vi "Periodic Tasks.vi"(8 "error in":errorcluster) -> ()   [LabVIEW 2018]
doc: "This VI runs in parallel to other tasks. It can contain as many user-defined periodic loops as you need. These can carry out PID or other sorts of timed response."
uses:
  <vilib>/Platform/TimedLoop/XDataNode/timing_clust.ctl
  <vilib>/Platform/TimedLoop/XDataNode/nitl_modes.ctl
  <vilib>/Platform/TimedLoop/XDataNode/wakeup.ctl
  <vilib>/Rock Robotics/WPI/ThirdParty/Phoenix-LabVIEW/Motor Controller/Controls/CTRE_Phoenix_MotorControl_ControlMode.ctl
  <vilib>/Rock Robotics/WPI/Utilities/WPI_GetSetVariantRefNum.vi
  <vilib>/Rock Robotics/WPI/Joystick/WPI_JoystickArcadeMapping.vi
  <vilib>/addons/control/pid/pid.llb/PID (DBL).vi
  <vilib>/addons/control/pid/pid.llb/PID Output Rate Limiter (DBL).vi
  <vilib>/platform/TimedLoop/XDataNode/XDataNode.xnode
  <vilib>/addons/control/pid/NI_PID_pid.lvlib
  <vilib>/Platform/TimedLoop/XDataNode/XDNodeRunTimeDep.lvlib
panel:
  in  "ms to wait":u32=50
  in  "Tab Control":enum32{"Auto Tape Alignment", "Drive PID Tune"}(tab)
  out "Late?":bool
  out "Arrived":bool
  in  "Tol (cnts)":dbl=10.0
  in  "Tol (sec)":dbl=0.25 format="%#_13g"
  in  "Approach":dbl=0.55 format="%#_13g"
  out "Value 1":bool
  out "Value 2":bool
  out "Value 4":bool
  in  "PID gains":T1={"proportional gain (Kc)"=0.005, "integral time (Ti, min)"=0.007, "derivative time (Td, min)"=0.001} {"derivative time (Td, min)" format="%.3f"; "integral time (Ti, min)" format="%.3f"; "proportional gain (Kc)" format="%.3f"}
  in  "clamp":cluster{"output high":dbl, "output low":dbl}={"output high"=0.8, "output low"=-0.8} {"output low" format="%.2f"; "output high" format="%.2f"}
  in  "Fwd offset":dbl=190.0
  in  "Rvs offset":dbl=150.0
  out "Goal":dbl=712.25
  out "Distance":dbl=364.5
  in  "rate":dbl=500.0 format="%.2f"
  out "Tape Width":dbl=34.5
  out "State":i32
  out "Error":dbl=347.75
  out "Align Assist":bool
  in  "Set":dbl(slide)=1.5948963317384823 scale=-1000.0..1000.0
  in  "output range":cluster{"output high":dbl, "output low":dbl}={"output high"=0.8, "output low"=-0.8} {"output low" format="%.2f"; "output high" format="%.2f"}
  in  "PID gains 2":T1={"proportional gain (Kc)"=0.005, "integral time (Ti, min)"=0.007, "derivative time (Td, min)"=0.001} {"derivative time (Td, min)" format="%.3f"; "integral time (Ti, min)" format="%.3f"; "proportional gain (Kc)" format="%.3f"}
  out "PID":cluster{"Set":dbl, "Distance":dbl}(graph)={"Set"=-687.4003189792663, "Distance"=-688.5}
  in  "output rate (EGU/min)":dbl=100.0 format="%.2f"
  out "Distance 2":dbl=-688.5
  out "Error 2":dbl=1.0996810207336694
  out "Motor":dbl=0.010401644622641346 format="%.2f"
  in  "Reset":bool
  in  "reinitialize? (F)":bool
  in  "negate":bool=TRUE
  out "Arrived 2":bool=TRUE
  in  "Tol 2":dbl=10.0
  # "Larger values move goal\nfurther in direction of travel"
  # "2016 Bot values:\nP=0.005, I=0.007, D=0.001"
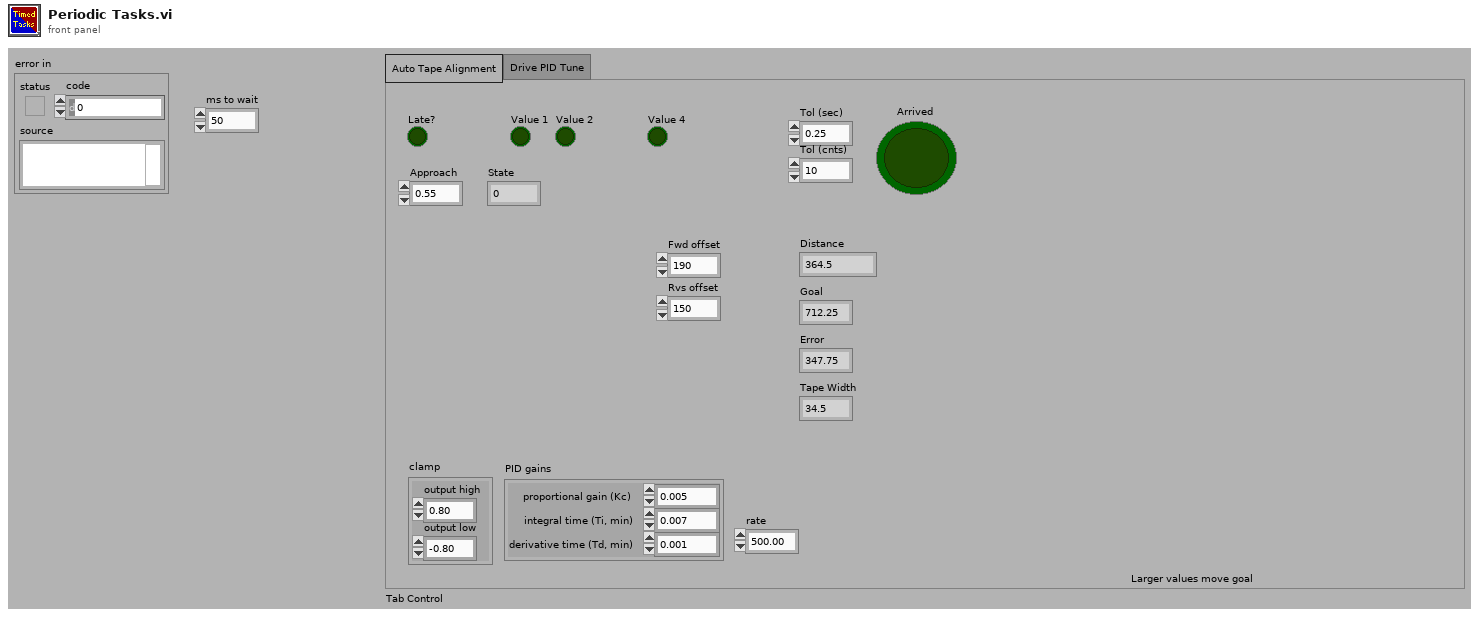
[diagram p1: front panel]
types:
  T1 = cluster{"proportional gain (Kc)":dbl, "integral time (Ti, min)":dbl, "derivative time (Td, min)":dbl}
  T2 = typedef "WPI_EncoderDevRef.ctl" = cluster{"DevStatus":errorcluster, "EncoderIndex":T3, "CounterIndex":T4, "DistancePerCount":dbl, "Decoding Type":T5}
  T3 = typedef "FPGA_EncoderIdx.ctl" = enum8{"Enc 0", "Enc 1", "Enc 2", "Enc 3", "Enc 4", "Enc 5", "Enc 6", "Enc 7", "Invalid"}
  T4 = typedef "FPGA_CounterCtrSystemIndex.ctl" = enum8{"Ctr 0", "Ctr 1", "Ctr 2", "Ctr 3", "Ctr 4", "Ctr 5", "Ctr 6", "Ctr 7", "Invalid"}
  T5 = typedef "WPI_EncoderType.ctl" = enum16{"1x", "2x", "4x"}
  T6 = typedef "WPI_DigitalInputDevRef.ctl" = cluster{"DevStatus":errorcluster, "DIO Channel":T7}
  T7 = typedef "FPGA_DIOChannel.ctl" = enum8{"DIO 0", "DIO 1", "DIO 2", "DIO 3", "DIO 4", "DIO 5", "DIO 6", "DIO 7", "DIO 8", "DIO 9", "DIO MXP 0", "DIO MXP 1", "DIO MXP 2", "DIO MXP 3", "DIO MXP 4", "DIO MXP 5", "DIO MXP 6", "DIO MXP 7", "DIO MXP 8", "DIO MXP 9", "DIO MXP 10", "DIO MXP 11", "DIO MXP 12", "DIO MXP 13", "DIO MXP 14", "DIO MXP 15", "SPI Port CS1", "SPI Port CS2", "SPI Port CS3", "SPI Port MISO", "SPI Port MOSI", "Invalid"}
  T8 = typedef "WPI_MotorControlDeviceRef.ctl" = cluster{"DeviceStatus":errorcluster, "Type":T9, "PWM":cluster{"PWM Channel":T10, "DeadBand":T11}, "CAN":cluster{"Device Number":u8, "SetOutput VI Ref":variant, "GetOutput VI Ref":variant, "Enable VI Ref":variant, "Disable VI Ref":variant, "Data":variant}, "Invert":bool, "DIO PWM":cluster{"PWM \"Enable\" Channel":T10, "DIOChannel":T7, "PWM Rate":dbl}}
  T9 = typedef "WPI_MotorControlType.ctl" = enum16{"PWM", "CAN", "DIO PWM"}
  T10 = typedef "FPGA_DIOPWMChannel.ctl" = enum8{"PWM 0", "PWM 1", "PWM 2", "PWM 3", "PWM 4", "PWM 5", "PWM 6", "PWM 7", "PWM 8", "PWM 9", "PWM MXP 0", "PWM MXP 1", "PWM MXP 2", "PWM MXP 3", "PWM MXP 4", "PWM MXP 5", "PWM MXP 6", "PWM MXP 7", "PWM MXP 8", "PWM MXP 9", "Invalid"}
  T11 = typedef "WPI_PWMDeadband.ctl" = cluster{"Name":string, "maxPositivePwm":i32, "minPositivePwm":i32, "centerPwm":i32, "maxNegativePwm":i32, "minNegativePwm":i32, "angularRange":u16}
  T12 = typedef "WPI_JoystickDevRef.ctl" = cluster{"Device":T13}
  T13 = typedef "WPI_JoystickDeviceEnum.ctl" = enum16{"USB 0", "USB 1", "USB 2", "USB 3", "USB 4", "USB 5"}
  T14 = typedef "XDNodeRunTimeDep.lvlib/timing_clust.ctl" = cluster{"Expected End [f-1]":u64, "Actual End [f-1]":u64, "Finished Late? [f-1]":bool, "Expected End [i-1]":u64, "Actual End [i-1]":u64, "Finished Late? [i-1]":bool, "Expected Start [i]":u64, "Actual Start [i]":u64, "Expected Start [f]":u64, "Actual Start [f]":u64, "Source Name":string, "Structure Name":string, "Period":i64, "Deadline":i64, "Offset":i64, "Start":i64, "Priority":i32, "Timeout":i32, "Mode":T15, "Wakeup Reason":T16, "Error":errorcluster, "Source Type":string, "Secondary Source Type":string, "Global End Time":u64, "Global Start Time":u64, "Frame Duration":u64, "Iteration Duration":u64, "Assigned CPU":i32, "I/O Scan Engine Mode":u32}
  T15 = typedef "XDNodeRunTimeDep.lvlib/nitl_modes.ctl" = enum32{"No Change", "Process missed periods, maintain original phase", "Discard missed periods, maintain original phase", "Process missed periods, ignore original phase", "Discard missed periods, ignore original phase"}
  T16 = typedef "XDNodeRunTimeDep.lvlib/wakeup.ctl" = enum32{"Normal", "Aborted", "Asynchronous wakeup", "Timing source error", "Timed loop error", "Timeout"}
  T17 = typedef "CTRE_Phoenix_MotorControl_ControlMode.ctl" = u16
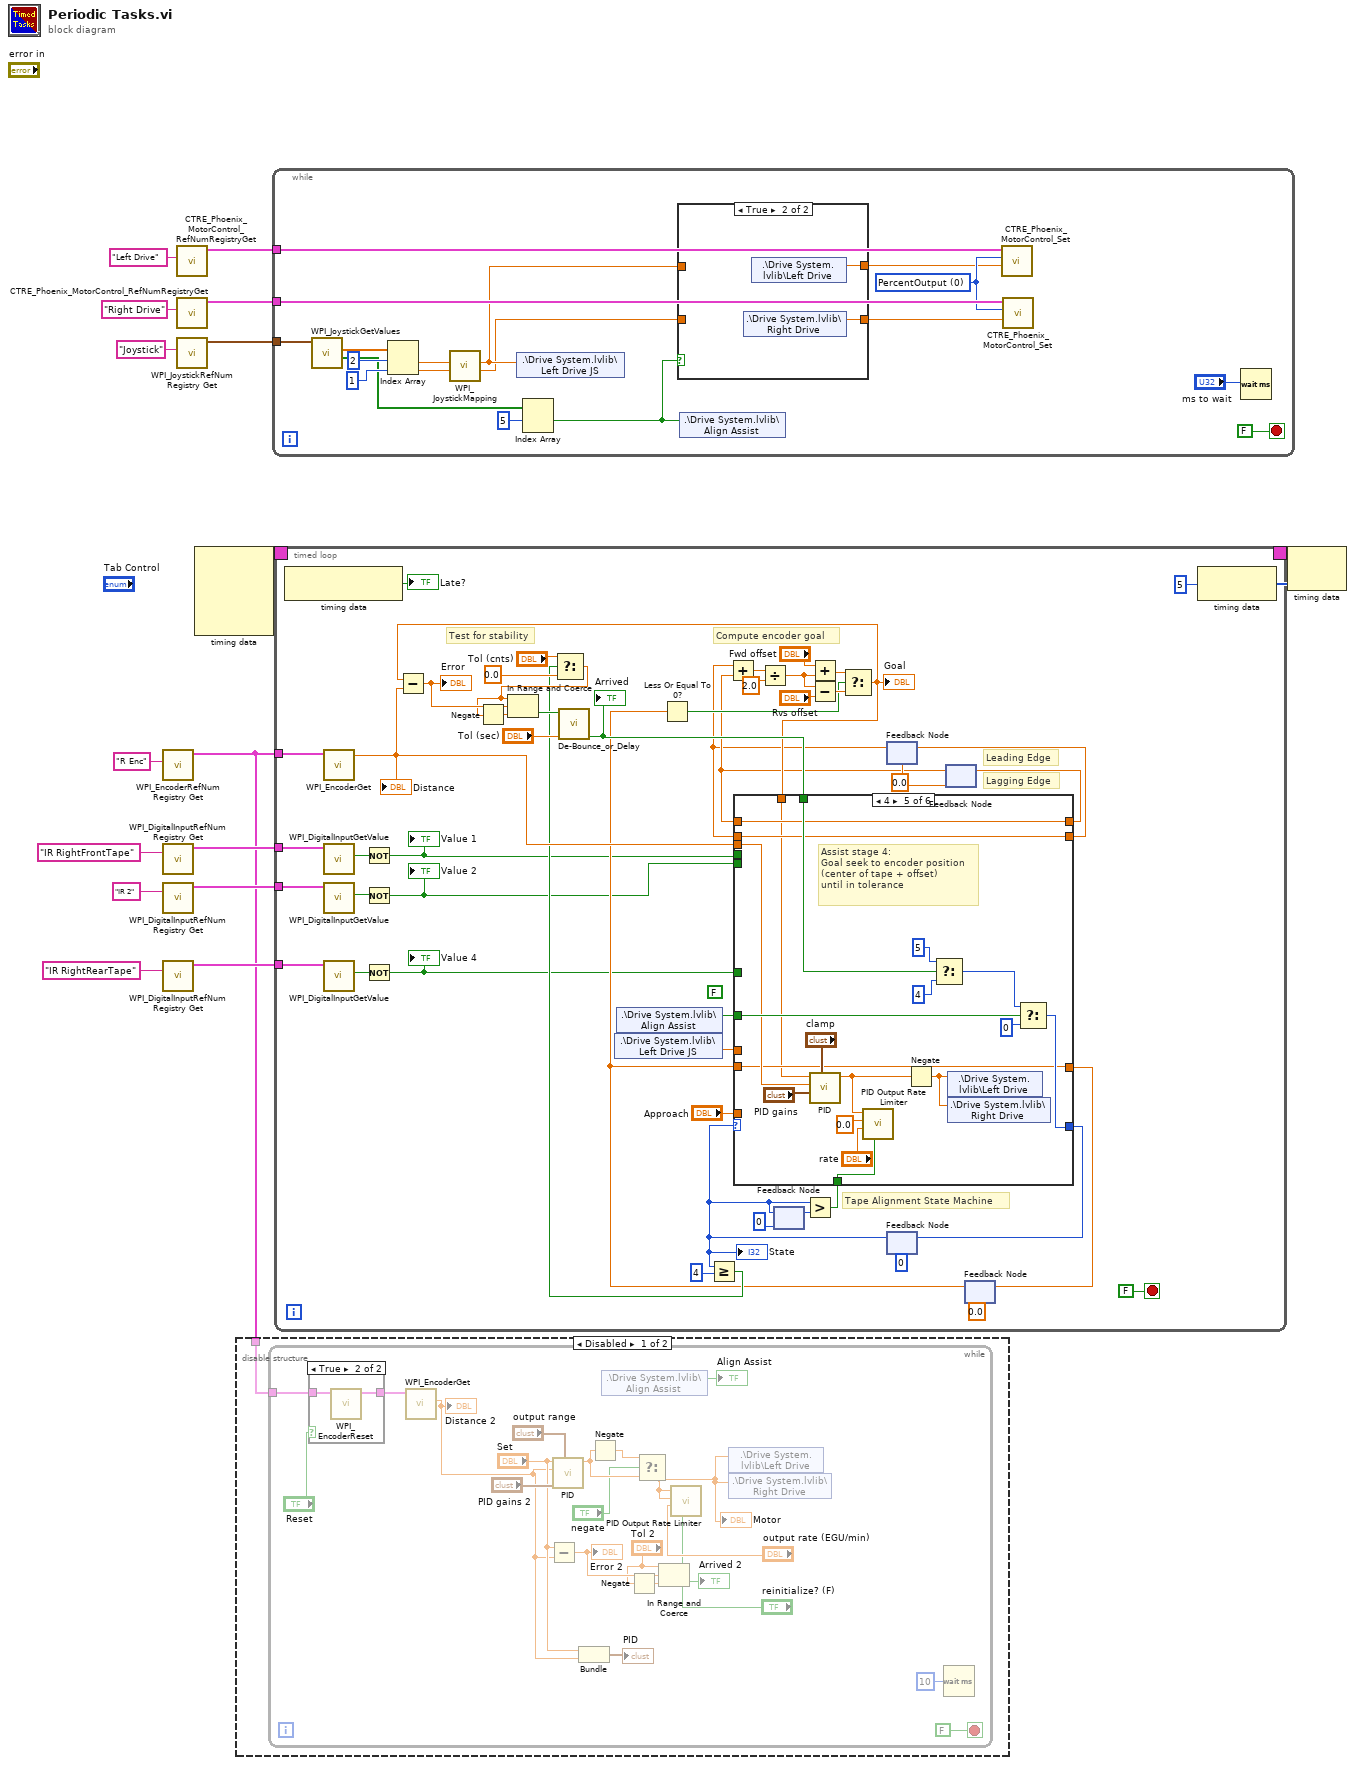
[diagram p0: block diagram]
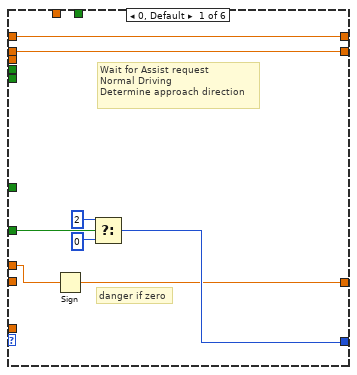
[diagram p2: hidden frame]
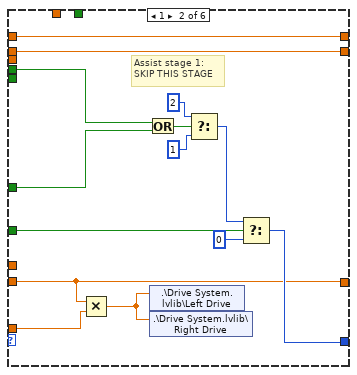
[diagram p3: hidden frame]
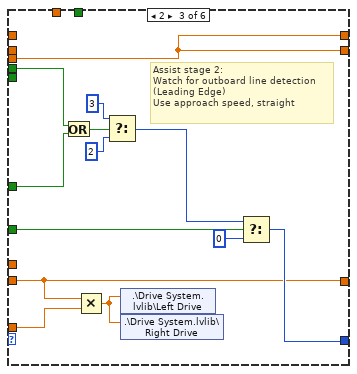
[diagram p4: hidden frame]
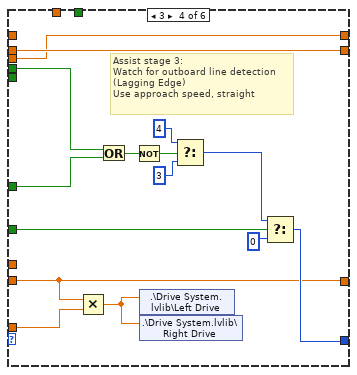
[diagram p5: hidden frame]
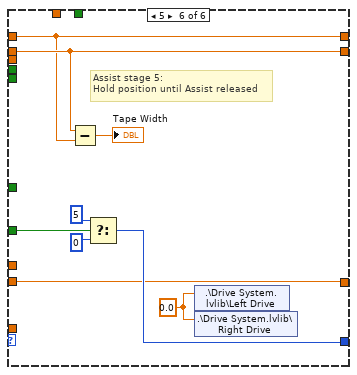
[diagram p6: hidden frame]
diagram:
  n1 = call <vilib>:"WPI_EncoderRefNum Registry Get.vi"("refnum name"="R Enc") -> ("EncoderDevRef"=w3:T2)  [unwired: 9 in, 1 out]
  n2 = call <vilib>:"WPI_DigitalInputRefNum Registry Get.vi"("refnum name"="IR RightFrontTape") -> ("DigitalInputDevRef"=w10:T6)  [unwired: 9 in, 1 out]
  n3 = call <vilib>:"WPI_DigitalInputRefNum Registry Get.vi"("refnum name"="IR 2") -> ("DigitalInputDevRef"=w9:T6)  [unwired: 9 in, 1 out]
  n4 = call <vilib>:"WPI_DigitalInputRefNum Registry Get.vi"("refnum name"="IR RightRearTape") -> ("DigitalInputDevRef"=w8:T6)  [unwired: 9 in, 1 out]
  n5 = call <vilib>:"CTRE_Phoenix_MotorControl_RefNumRegistryGet.vi"("refnum name"="Left Drive") -> ("PhoenixMotorControlDevRef"=w12:T8)  [unwired: 9 in, 1 out]
  n6 = call <vilib>:"CTRE_Phoenix_MotorControl_RefNumRegistryGet.vi"("refnum name"="Right Drive") -> ("PhoenixMotorControlDevRef"=w11:T8)  [unwired: 9 in, 1 out]
  n7 = call <vilib>:"WPI_JoystickRefNum Registry Get.vi"("refnum name"="Joystick") -> ("JoystickDevRef"=w14:T12)  [unwired: 1 in, 9 out]
  n8 = node-c288() -> (w2:T14)  [unwired: 4 in]
  n9 = disable-structure shown="Disabled" {
    disable-tunnel: w3 -> [w17 _]
    frame Disabled {
      n10 = while {
        tunnel: w17 -> [w27]
        stop <- FALSE stop-if-true
        n11 = case shown="True" "Reset" {
          tunnel: w27 -> [w39 w41]
          tunnel: [w39 w40] -> w26
          frame False {
          }
          frame True {
            n12 = call <vilib>:"WPI_EncoderReset.vi"("EncoderDevRef"=w41) -> ("EncoderDevRef"=w40:T2)  [unwired: 9 in, 1 out]
          }
        }
        n13 = call <vilib>:"WPI_EncoderGet.vi"("EncoderDevRef"=w26) -> ("Distance"=w29:dbl)  [unwired: 5 in, 5 out]
        "Distance 2" <- w29
        n14 = Subtract(x="Set", y=w29) -> (x-y=w25:dbl)
        "Error 2" <- w25
        n15 = call-poly <vilib>:"PID.vi"("output range"="output range", "PID gains"="PID gains 2", "process variable"=w29, "setpoint"="Set") -> ("output"=w33:dbl)  [unwired: 6 in, 1 out]
        n16 = Bundle("Set"="Set", "Distance"=w29) -> (→"PID":cluster{"Set":dbl, "Distance":dbl})  [unwired: 1 in]
        n17 = Negate(x=w33) -> (-x=w32:dbl)
        n18 = shared-variable ".\\Drive System.lvlib\\Align Assist"() -> (→"Align Assist":bool)  [unwired: 1 in, 1 out]
        n19 = Negate(x="Tol 2") -> (-x=w23:dbl)
        n20 = Select(t=w32, s="negate", f=w33) -> (s? t:f=w18:dbl)
        "Motor" <- w18
        n21 = In Range and Coerce(upper limit="Tol 2", x=w25, lower limit=w23) -> (In Range?=→"Arrived 2":bool)  [unwired: 1 out]
        n22 = call-poly <vilib>:"PID Output Rate Limiter.vi"("reinitialize? (F)"="reinitialize? (F)", "output rate (EGU/min)"="output rate (EGU/min)", "initial output"=w18, "input (controller output)"=w18) -> ()  [unwired: 4 in, 2 out]
        n23 = shared-variable ".\\Drive System.lvlib\\Left Drive"(w18) -> ()  [unwired: 1 in, 1 out]
        n24 = shared-variable ".\\Drive System.lvlib\\Right Drive"(w18) -> ()  [unwired: 1 in, 1 out]
        n25 = Wait (ms)(milliseconds to wait=u32 10) -> ()  [unwired: 1 out]
      }
    }
    frame Enabled {
    }
  }
  n26 = while {
    tunnel: w14 -> [w59]
    tunnel: w12 -> [w53]
    tunnel: w11 -> [w52]
    stop <- FALSE stop-if-true
    w51 = T17 0 items=["PercentOutput"=0, "Position"=1, "Velocity"=2, "Current"=3, "Follower"=5, "MotionProfile"=6, "MotionMagic"=7, "MotionProfileArc"=10, "Disabled"=15] ("Control Mode")
    n27 = call <vilib>:"WPI_JoystickGetValues.vi"("JoystickDevRef"=w59) -> ("Buttons"=w49:bool[], "Axes"=w57:dbl[])  [unwired: 6 in, 3 out]
    n28 = Index Array(array=w57, index #1=2 ("index"), index #2=1 ("index")) -> (element #1=w55:dbl, element #2=w54:dbl)
    n29 = call-poly <vilib>:"WPI_JoystickMapping.vi"("Y axis value"=w54, "X axis value"=w55) -> ("Right Motor Value"=w43:dbl, "Left Motor Value"=w45:dbl)  [unwired: 8 in]
    n30 = shared-variable ".\\Drive System.lvlib\\Left Drive JS"(w45) -> ()  [unwired: 1 in, 1 out]
    n31 = Index Array(array=w49, index #1=5 ("index")) -> (element #1=w46:bool)  [unwired: 1 in, 1 out]
    n32 = case shown="True" w46 {
      tunnel: [w61 w63] -> w44
      tunnel: w45 -> [w61 _]
      tunnel: [w60 w62] -> w42
      tunnel: w43 -> [w60 _]
      frame False {
      }
      frame True {
        n33 = shared-variable ".\\Drive System.lvlib\\Right Drive"() -> (w62:dbl)  [unwired: 1 in, 1 out]
        n34 = shared-variable ".\\Drive System.lvlib\\Left Drive"() -> (w63:dbl)  [unwired: 1 in, 1 out]
      }
    }
    n35 = shared-variable ".\\Drive System.lvlib\\Align Assist"(w46) -> ()  [unwired: 1 in, 1 out]
    n36 = call <vilib>:"CTRE_Phoenix_MotorControl_Set.vi"("Output"=w44, "Control Mode"=w51, "PhoenixMotorControlDevRef"=w53) -> ()  [unwired: 7 in, 2 out]
    n37 = call <vilib>:"CTRE_Phoenix_MotorControl_Set.vi"("Output"=w42, "Control Mode"=w51, "PhoenixMotorControlDevRef"=w52) -> ()  [unwired: 7 in, 2 out]
    n38 = Wait (ms)(milliseconds to wait="ms to wait") -> ()  [unwired: 1 out]
  }
  n39 = timed-loop {
    tunnel: w10 -> [w113]
    tunnel: w9 -> [w112]
    tunnel: w8 -> [w111]
    tunnel: w3 -> [w103]
    timing: w2 -> [_]
    timing-out: [_] -> w1
    stop <- FALSE stop-if-true
    (unwired) FALSE ("Boolean")
    w83 = 0.0 ("Distance")
    # "Tape Alignment State Machine"
    # "Compute encoder goal"
    # "Test for stability"
    # "Lagging Edge"
    # "Leading Edge"
    n40 = node-c288() -> (→"Late?":bool)  [unwired: 1 in]
    n41 = call <vilib>:"WPI_EncoderGet.vi"("EncoderDevRef"=w103) -> ("Distance"=w98:dbl)  [unwired: 5 in, 5 out]
    "Distance" <- w98
    n42 = call <vilib>:"WPI_DigitalInputGetValue.vi"("DigitalInputDevRef"=w113) -> ("Value"=w109:bool)  [unwired: 8 in, 2 out]
    n43 = call <vilib>:"WPI_DigitalInputGetValue.vi"("DigitalInputDevRef"=w112) -> ("Value"=w108:bool)  [unwired: 8 in, 2 out]
    n44 = call <vilib>:"WPI_DigitalInputGetValue.vi"("DigitalInputDevRef"=w111) -> ("Value"=w107:bool)  [unwired: 8 in, 2 out]
    n45 = Not(x=w109) -> (.not. x?=w68:bool)
    "Value 1" <- w68
    n46 = Not(x=w108) -> (.not. x?=w67:bool)
    "Value 2" <- w67
    n47 = Not(x=w107) -> (.not. x?=w66:bool)
    "Value 4" <- w66
    n48 = shared-variable ".\\Drive System.lvlib\\Left Drive JS"() -> (w105:dbl)  [unwired: 1 in, 1 out]
    n49 = shared-variable ".\\Drive System.lvlib\\Align Assist"() -> (w80:bool)  [unwired: 1 in, 1 out]
    n50 = feedback #1(0) -> (w96:i32)
    n51 = feedback #2(w83) -> (w64:dbl)
    n52 = feedback #3(0) -> (w87:i32)
    "State" <- w87
    n53 = Greater Or Equal?(x=w87, y=4) -> (x >= y?=w85:bool)
    n54 = Select(t="Tol (cnts)", s=w85, f=0.0 ("t")) -> (s? t:f=w90:dbl)
    n55 = Negate(x=w90) -> (-x=w100:dbl)
    n56 = feedback-in #1(w87) -> ()
    n57 = Greater?(x=w87, y=w96) -> (0:w94:bool)
    n58 = feedback #4(w83) -> (w65:dbl)
    n59 = Add(x=w64, y=w65) -> (x+y=w73:dbl)
    n60 = Divide(x=w73, y=2.0) -> (x/y=w75:dbl)
    n61 = Add(x="Fwd offset", y=w75) -> (x+y=w78:dbl)
    n62 = Subtract(x=w75, y="Rvs offset") -> (x-y=w79:dbl)
    n63 = feedback #5(0.0) -> (w71:dbl)
    n64 = Less Or Equal To 0?(x=w71) -> (x <= 0?=w72:bool)
    n65 = Select(t=w78, s=w72, f=w79) -> (s? t:f=w74:dbl)
    "Goal" <- w74
    n66 = Subtract(x=w74, y=w98) -> (x-y=w101:dbl)
    "Error" <- w101
    n67 = In Range and Coerce(upper limit=w90, x=w101, lower limit=w100) -> (In Range?=w92:bool)  [unwired: 1 out]
    n68 = call <userlib>:"De-Bounce_or_Delay.vi"("Eval Period (sec)"="Tol (sec)", "Signal Input"=w92) -> ("Stable"=w91:bool)  [unwired: 9 in]
    "Arrived" <- w91
    n69 = case shown="4" w87 {
      tunnel: [w123 w137 w151 w166 w183 w193] -> w97
      tunnel: w80 -> [w126 w136 w150 w168 w182 w196]
      tunnel: w105 -> [w122 _ _ _ _ _]
      tunnel: [w121 w133 w147 w160 w171 w192] -> w106
      tunnel: w71 -> [_ w133 w147 w160 w171 w192]
      tunnel: w66 -> [_ w132 w143 w157 _ _]
      tunnel: w68 -> [_ w131 w144 w155 _ _]
      tunnel: w67 -> [_ _ _ _ _ _]
      tunnel: w98 -> [_ _ w145 w162 w179 _]
      tunnel: [w120 w129 w145 w163 w173 w190] -> w102
      tunnel: w64 -> [w120 w129 _ w163 w173 w190]
      tunnel: w91 -> [_ _ _ _ w174 _]
      tunnel: w94 -> [_ _ _ _ w175 _]
      tunnel: [w119 w128 w145 w162 w172 w189] -> w84
      tunnel: w65 -> [w119 w128 _ _ w172 w189]
      tunnel: "Approach" -> [_ w127 w141 w154 _ _]
      tunnel: w74 -> [_ _ _ _ w169 _]
      frame 0, Default {
        # "Wait for Assist request\nNormal Driving\nDetermine approach direction"
        # "danger if zero"
        n70 = Sign(1:w122) -> (0:w121:dbl)
        n71 = Select(t=2, s=w126, f=0) -> (s? t:f=w123:i32)
      }
      frame 1 {
        # "Assist stage 1:\nSKIP THIS STAGE"
        n72 = Multiply(x=w133, y=w127) -> (x*y=w130:dbl)
        n73 = Or(x=w131, y=w132) -> (x .or. y?=w140:bool)
        n74 = shared-variable ".\\Drive System.lvlib\\Left Drive"(w130) -> ()  [unwired: 1 in, 1 out]
        n75 = shared-variable ".\\Drive System.lvlib\\Right Drive"(w130) -> ()  [unwired: 1 in, 1 out]
        n76 = Select(t=2, s=w140, f=1) -> (s? t:f=w135:i32)
        n77 = Select(t=w135, s=w136, f=0) -> (s? t:f=w137:i32)
      }
      frame 2 {
        # "Assist stage 2:\nWatch for outboard line detection\n(Leading Edge)\nUse approach speed, straight"
        n78 = Or(x=w144, y=w143) -> (x .or. y?=w142:bool)
        n79 = Multiply(x=w147, y=w141) -> (x*y=w146:dbl)
        n80 = Select(t=3 ("Jump"), s=w142, f=2) -> (s? t:f=w149:i32)
        n81 = shared-variable ".\\Drive System.lvlib\\Left Drive"(w146) -> ()  [unwired: 1 in, 1 out]
        n82 = shared-variable ".\\Drive System.lvlib\\Right Drive"(w146) -> ()  [unwired: 1 in, 1 out]
        n83 = Select(t=w149, s=w150, f=0) -> (s? t:f=w151:i32)
      }
      frame 3 {
        # "Assist stage 3:\nWatch for outboard line detection\n(Lagging Edge)\nUse approach speed, straight"
        n84 = Multiply(x=w160, y=w154) -> (x*y=w159:dbl)
        n85 = Or(x=w155, y=w157) -> (x .or. y?=w156:bool)
        n86 = Not(x=w156) -> (.not. x?=w158:bool)
        n87 = shared-variable ".\\Drive System.lvlib\\Left Drive"(w159) -> ()  [unwired: 1 in, 1 out]
        n88 = shared-variable ".\\Drive System.lvlib\\Right Drive"(w159) -> ()  [unwired: 1 in, 1 out]
        n89 = Select(t=4, s=w158, f=3) -> (s? t:f=w161:i32)
        n90 = Select(t=w161, s=w168, f=0) -> (s? t:f=w166:i32)
      }
      frame 4 {
        # "Assist stage 4:\nGoal seek to encoder position\n(center of tape + offset)\nuntil in tolerance"
        n91 = call-poly <vilib>:"PID.vi"("output range"="clamp", "PID gains"="PID gains", "process variable"=w179, "setpoint"=w169) -> ("output"=w170:dbl)  [unwired: 6 in, 1 out]
        n92 = call-poly <vilib>:"PID Output Rate Limiter.vi"("reinitialize? (F)"=w175, "output rate (EGU/min)"="rate", "initial output"=0.0, "input (controller output)"=w170) -> ()  [unwired: 4 in, 2 out]
        n93 = Negate(x=w170) -> (-x=w181:dbl)
        n94 = Select(t=5, s=w174, f=4) -> (s? t:f=w184:i32)
        n95 = shared-variable ".\\Drive System.lvlib\\Left Drive"(w181) -> ()  [unwired: 1 in, 1 out]
        n96 = shared-variable ".\\Drive System.lvlib\\Right Drive"(w181) -> ()  [unwired: 1 in, 1 out]
        n97 = Select(t=w184, s=w182, f=0) -> (s? t:f=w183:i32)
      }
      frame 5 {
        w191 = 0.0 ("Slow 2")
        # "Assist stage 5:\nHold position until Assist released"
        n98 = Subtract(x=w190, y=w189) -> (x-y=→"Tape Width":dbl)
        n99 = Select(t=5, s=w196, f=0) -> (s? t:f=w193:i32)
        n100 = shared-variable ".\\Drive System.lvlib\\Left Drive"(w191) -> ()  [unwired: 1 in, 1 out]
        n101 = shared-variable ".\\Drive System.lvlib\\Right Drive"(w191) -> ()  [unwired: 1 in, 1 out]
      }
    }
    n102 = feedback-in #2(w102) -> ()
    n103 = feedback-in #3(w97) -> ()
    n104 = feedback-in #4(w84) -> ()
    n105 = feedback-in #5(w106) -> ()
    n106 = node-c288(i64 5 ("Period")) -> ()  [unwired: 1 out]
  }
  n107 = node-c288(w1) -> ()  [unwired: 1 out]
